vi "Troubleshooting and Debugging VIs.vi"() -> ()   [LabVIEW 2022 SP3]
panel:
  out "Numeric 3":dbl
  in  "Numeric 2":dbl
  in  "Numeric":dbl
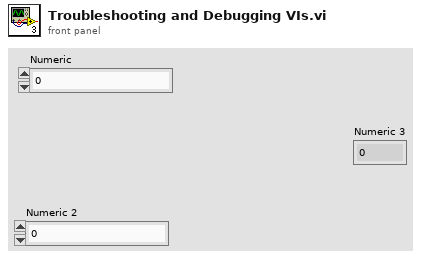
[diagram p1: front panel]
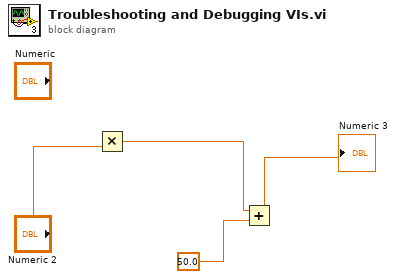
[diagram p0: block diagram]
diagram:
  n1 = Multiply(y="Numeric 2") -> (x*y=w3:dbl)  [unwired: 1 in]
  n2 = Add(x=w3, y=50.0) -> (x+y=→"Numeric 3":dbl)
